vi "GetGlobalDefaultConfiguration.vi"(3 "Read defaults?":bool) -> (1 "Configuration File IV":path)   [LabVIEW 2013]
uses:
  MeasurementSetup.vi
panel:
  out "Configuration File Cis":path
  out "Configuration File Stability":path
  out "Configuration File CV":path
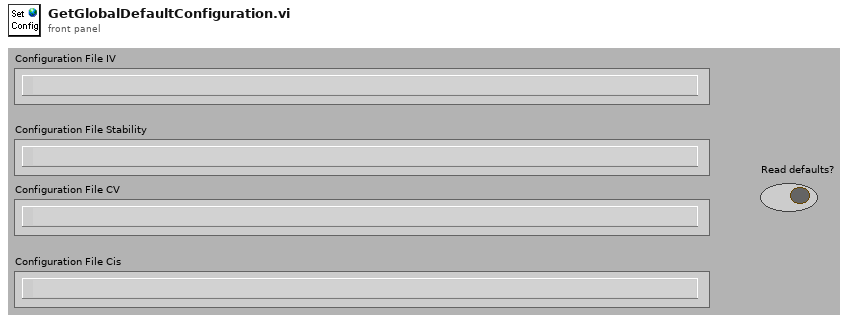
[diagram p1: front panel]
types:
  T1 = cluster{"Supply":refnum<class "SupplyControl.lvclass">, "Initial Voltage [V]":dbl, "Final Voltage [V]":dbl, "Step Size [V]":dbl, "Step Interval [s]":i32, "Number Of Steps":u32, "Ramp down steps [V]":dbl, "Ramp down Interval [s]":i32, "Set Current Limit?":bool, "Current Limit [µA]":dbl, "Temperature Readout":enum16{"Read Arduino", "Enter manually"}, "Arduino":refnum<class "ArduinoControl.lvclass">, "Supply Name":string}
  T2 = cluster{"Supply":refnum<class "SupplyControl.lvclass">, "LCR":refnum<class "LCRControl.lvclass">, "Initial Voltage [V]":dbl, "Final Voltage [V]":dbl, "Step Size [V]":dbl, "Step Interval [s]":i32, "Number Of Steps":u32, "AC frequency [Hz]":i32, "RC Configuration":u16, "AC amplitude [V]":dbl, "Ramp down steps [V]":dbl, "Ramp down Delay [s]":i32, "Set Current Limit?":bool, "Current Limit [µA]":dbl, "Temperature Readout":enum16{"Read Arduino", "Enter manually"}, "Arduino":refnum<class "ArduinoControl.lvclass">, "Supply Name":string, "LCR Name":string}
  T3 = cluster{"Supply":refnum<class "SupplyControl.lvclass">, "Voltage [V]":dbl, "Measurement Interval [s]":i32, "Test Duration":u32, "Ramp up steps [V]":dbl, "Ramp up Interval [s]":u32, "Ramp down steps [V]":dbl, "Ramp down Interval [s]":i32, "Set Current Limit?":bool, "Current Limit [µA]":dbl, "Temperature Readout":enum16{"Read Arduino", "Enter manually"}, "Arduino":refnum<class "ArduinoControl.lvclass">, "Supply Name":string}
  T4 = cluster{"Supply":refnum<class "SupplyControl.lvclass">, "LCR":refnum<class "LCRControl.lvclass">, "Initial Voltage [V]":dbl, "Final Voltage [V]":dbl, "Step Size [V]":dbl, "Step Interval [s]":i32, "Number Of Steps":u32, "AC frequency [Hz]":i32, "RC Configuration":u16, "AC amplitude [V]":dbl, "Ramp down steps [V]":dbl, "Ramp down Interval [s]":i32, "Set Current Limit?":bool, "Current Limit [µA]":dbl, "Temperature Readout":enum16{"Read Arduino", "Enter manually"}, "Arduino":refnum<class "ArduinoControl.lvclass">, "Supply Name":string, "LCR Name":string}
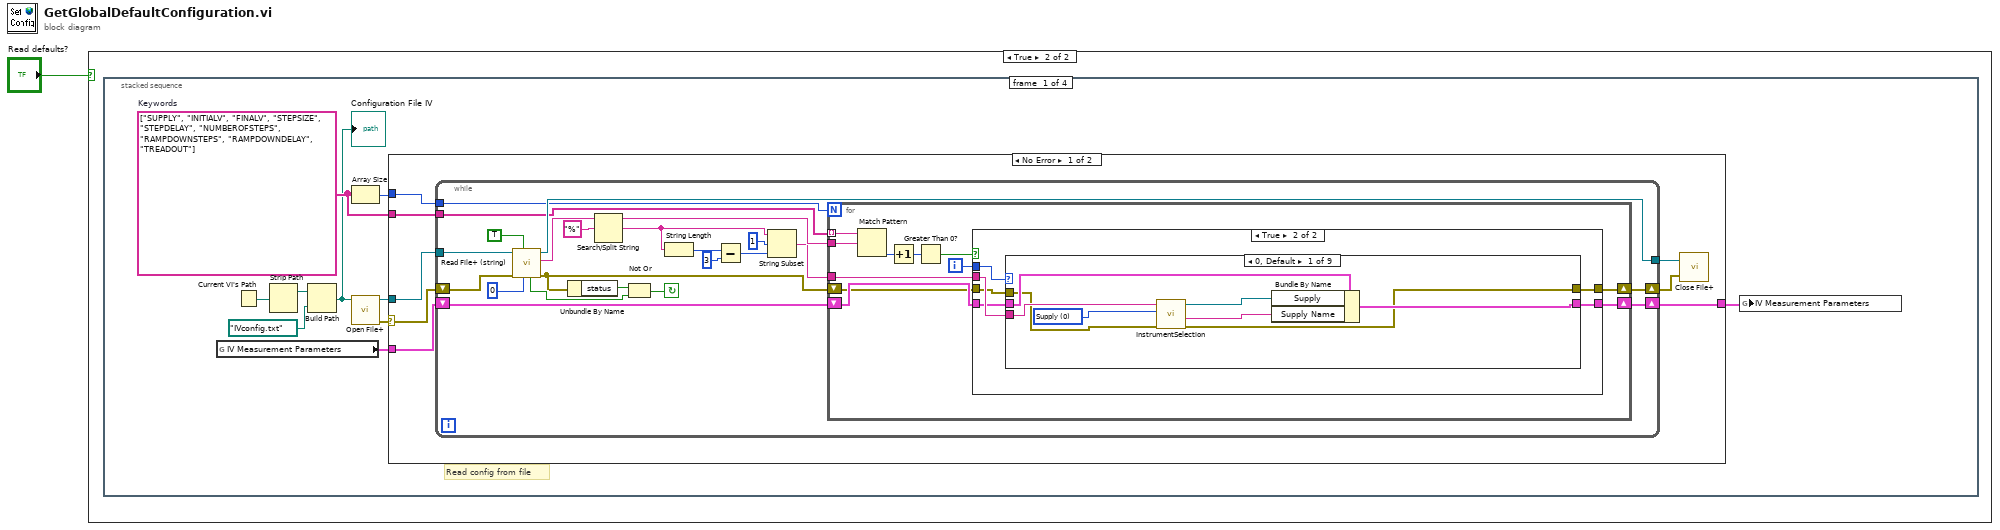
[diagram p0: block diagram]
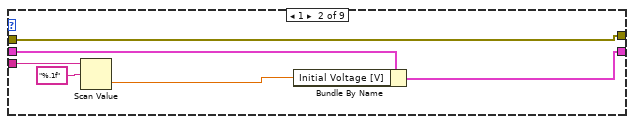
[diagram p4: hidden frame]
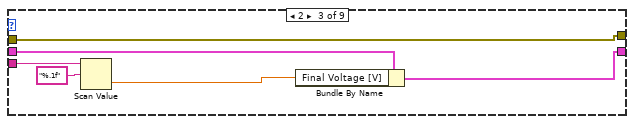
[diagram p5: hidden frame]
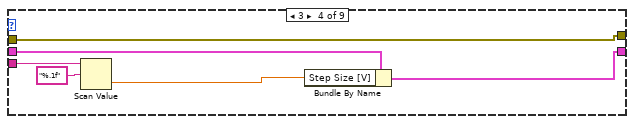
[diagram p6: hidden frame]
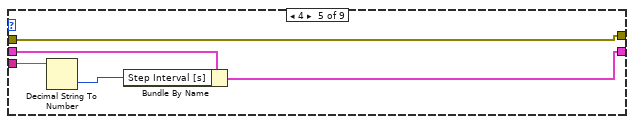
[diagram p7: hidden frame]
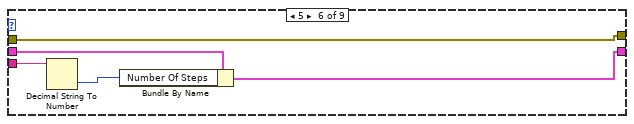
[diagram p8: hidden frame]
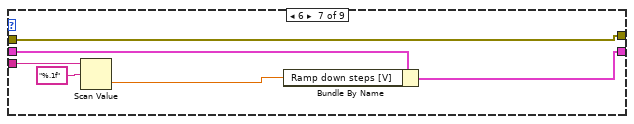
[diagram p9: hidden frame]
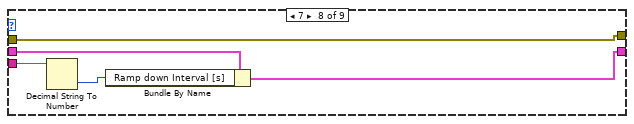
[diagram p10: hidden frame]
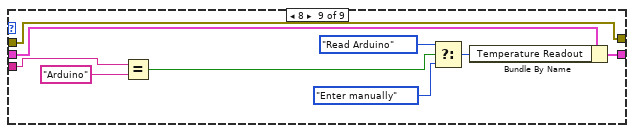
[diagram p11: hidden frame]
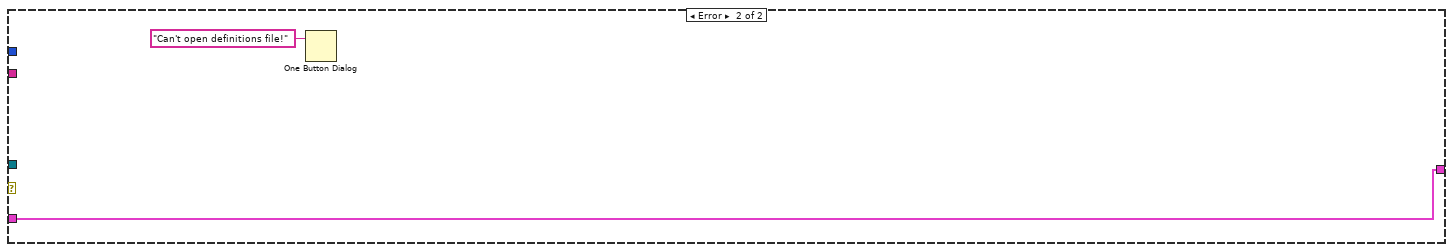
[diagram p12: hidden frame]
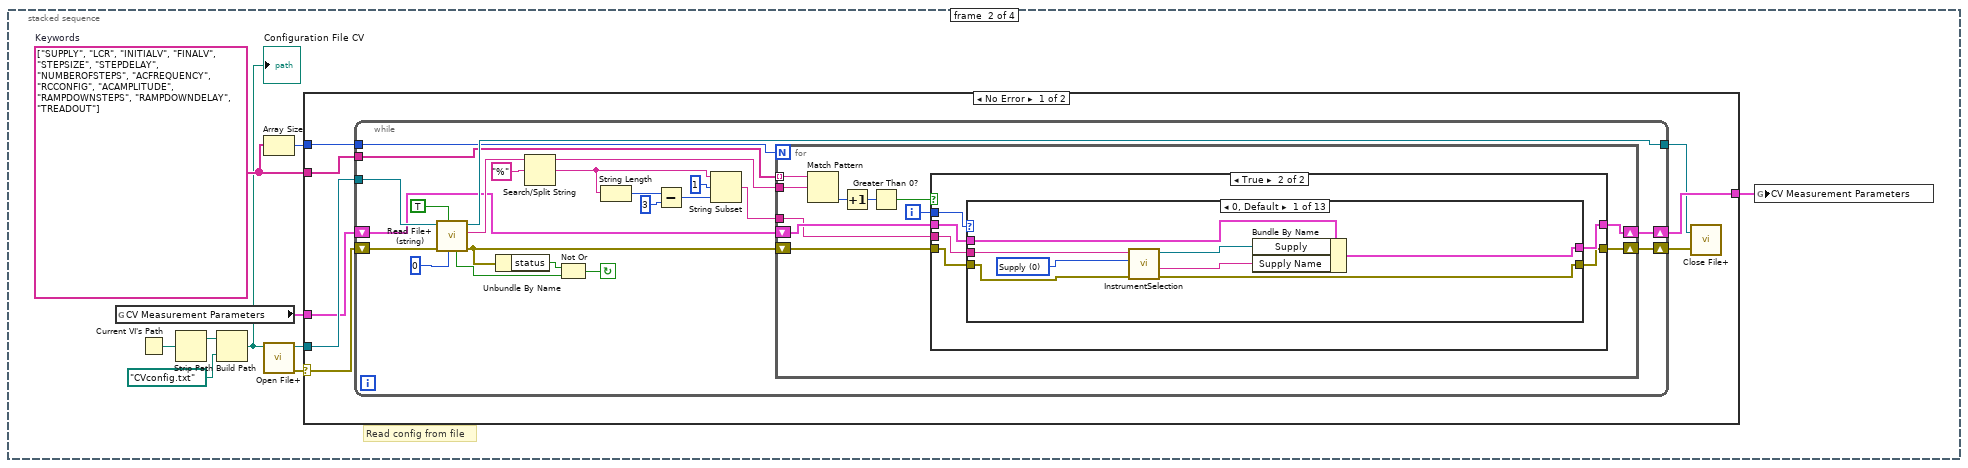
[diagram p13: hidden frame]
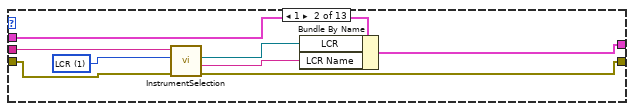
[diagram p15: hidden frame]
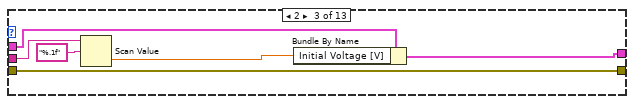
[diagram p16: hidden frame]
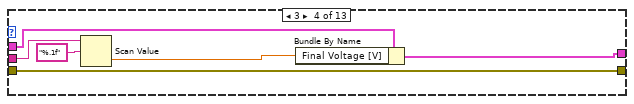
[diagram p17: hidden frame]
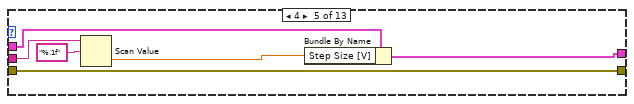
[diagram p18: hidden frame]
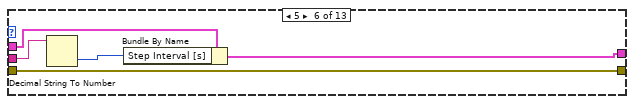
[diagram p19: hidden frame]
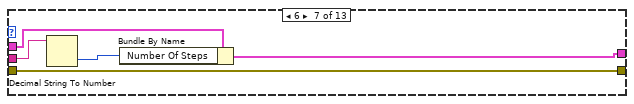
[diagram p20: hidden frame]
diagram:
  n1 = case shown="True" "Read defaults?" {
    frame False {
    }
    frame True {
      n2 = stacked-sequence {
        frame #0 {
          w11 = string[] ["SUPPLY", "INITIALV", "FINALV", "STEPSIZE", "STEPDELAY", "NUMBEROFSTEPS", "RAMPDOWNSTEPS", "RAMPDOWNDELAY", "TREADOUT"]  # Keywords
          # "Read config from file"
          n3 = global read "MeasurementSetup.vi" "IV Measurement Parameters"() -> (w2:T1)
          n4 = Current VI's Path() -> (path=w6:path)
          n5 = Strip Path(path=w6) -> (stripped path=w5:path)  [unwired: 1 out]
          n6 = Build Path(base path=w5, name or relative path=path "IVconfig.txt") -> (appended path=w4:path)
          "Configuration File IV" <- w4
          n7 = Array Size(array=w11) -> (size(s)=w10:i32)
          n8 = call <vilib>:"Open File+.vi"("file path (\" \")"=w4) -> ("error out"=w7:errorcluster, "refnum"=w8:refnum<file>)  [unwired: 7 in, 2 out]
          n9 = case shown="No Error" w7 {
            selector: w7 -> [w12 _]
            tunnel: w8 -> [w19 _]
            tunnel: w11 -> [w18 _]
            tunnel: w10 -> [w17 _]
            tunnel: w2 -> [w16 w118]
            tunnel: [w15 w118] -> w3
            frame No Error {
              n10 = while {
                shift-left: w16 -> [w25]
                shift-right: [w23] -> w15
                tunnel: w17 -> [w22]
                tunnel: w18 -> [w28]
                tunnel: [w33] -> w14
                tunnel: w19 -> [w39]
                shift-right: [w20] -> w13
                shift-left: w12 -> [w32]
                stop <- w35 continue-if-true
                n11 = call <vilib>:"Read File+ (string).vi"("count"=0, "line mode (characters:F)"=TRUE, "error in (no error)"=w32, "refnum"=w39) -> ("error out"=w21:errorcluster, "string"=w34:string, "dup refnum"=w33:refnum<file>, "EOF?"=w37:bool)  [unwired: 3 in, 1 out]
                n12 = Unbundle By Name(w21) -> ("status"=w36:bool)
                n13 = Search/Split String(string=w34, search string/char (-)="%" ("search char (-)")) -> (substring before match=w27:string, match + rest of string=w40:string)  [unwired: 1 in, 1 out]
                n14 = Not Or(1:w37, 2:w36) -> (0:w35:bool)
                n15 = String Length(string=w40) -> (length=w26:i32)
                n16 = Subtract(x=w26, y=3) -> (x-y=w29:i32)
                n17 = String Subset(string=w40, offset (0)=1, length (rest)=w29) -> (substring=w24:string)
                n18 = for {
                  N: w22 -> [_]
                  tunnel: w28 -> [w51] mode=indexing
                  tunnel: w27 -> [w46]
                  shift-right: [w47] -> w23
                  shift-left: w25 -> [w48]
                  tunnel: w24 -> [w45]
                  shift-right: [w43] -> w20
                  shift-left: w21 -> [w44]
                  i -> [w49]
                  n19 = Match Pattern(string=w51, regular expression=w46) -> (offset past match=w52:i32)  [unwired: 1 in, 3 out]
                  n20 = Increment(x=w52) -> (x+1=w53:i32)
                  n21 = Greater Than 0?(x=w53) -> (x > 0?=w50:bool)
                  n22 = case shown="True" w50 {
                    tunnel: w49 -> [_ w61]
                    tunnel: w45 -> [_ w60]
                    tunnel: w48 -> [w55 w59]
                    tunnel: [w55 w58] -> w47
                    tunnel: w44 -> [w54 w57]
                    tunnel: [w54 w56] -> w43
                    frame False {
                    }
                    frame True {
                      n23 = case shown="0, Default" w61 {
                        tunnel: w60 -> [w66 w73 w78 w84 w90 w95 w100 w106 w115]
                        tunnel: w59 -> [w69 w75 w81 w87 w92 w97 w103 w108 w117]
                        tunnel: [w68 w74 w80 w86 w91 w96 w102 w107 w116] -> w58
                        tunnel: w57 -> [w65 w70 w76 w82 w88 w93 w98 w104 w109]
                        tunnel: [w64 w70 w76 w82 w88 w93 w98 w104 w109] -> w56
                        frame 0, Default {
                          w67 = u16 0 items=["Supply", "LCR"] ("Instrument type")
                          n24 = call "InstrumentSelection.vi"("error in (no error)"=w65, "Instrument type"=w67, "Instrument name IN"=w66) -> ("error out"=w64:errorcluster, "Instrument name OUT"=w63:string, "Supply"=w62:refnum<class "SupplyControl.lvclass">)  [unwired: 5 in, 1 out]
                          n25 = Bundle By Name(cluster=w69, "Supply"=w62, "Supply Name"=w63) -> (w68:T1)
                        }
                        frame 1 {
                          n26 = Scan Value(string=w73, format string="%.1f") -> (value=w72:dbl)  [unwired: 1 in, 1 out]
                          n27 = Bundle By Name(cluster=w75, "Initial Voltage [V]"=w72) -> (w74:T1)
                        }
                        frame 2 {
                          n28 = Scan Value(string=w78, format string="%.1f") -> (value=w77:dbl)  [unwired: 1 in, 1 out]
                          n29 = Bundle By Name(cluster=w81, "Final Voltage [V]"=w77) -> (w80:T1)
                        }
                        frame 3 {
                          n30 = Scan Value(string=w84, format string="%.1f") -> (value=w83:dbl)  [unwired: 1 in, 1 out]
                          n31 = Bundle By Name(cluster=w87, "Step Size [V]"=w83) -> (w86:T1)
                        }
                        frame 4 {
                          n32 = Decimal String To Number(string=w90) -> (number=w89:i32)  [unwired: 2 in, 1 out]
                          n33 = Bundle By Name(cluster=w92, "Step Interval [s]"=w89) -> (w91:T1)
                        }
                        frame 5 {
                          n34 = Decimal String To Number(string=w95) -> (number=w94:i32)  [unwired: 2 in, 1 out]
                          n35 = Bundle By Name(cluster=w97, "Number Of Steps"=w94) -> (w96:T1)
                        }
                        frame 6 {
                          n36 = Scan Value(string=w100, format string="%.1f") -> (value=w99:dbl)  [unwired: 1 in, 1 out]
                          n37 = Bundle By Name(cluster=w103, "Ramp down steps [V]"=w99) -> (w102:T1)
                        }
                        frame 7 {
                          n38 = Decimal String To Number(string=w106) -> (number=w105:i32)  [unwired: 2 in, 1 out]
                          n39 = Bundle By Name(cluster=w108, "Ramp down Interval [s]"=w105) -> (w107:T1)
                        }
                        frame 8 {
                          n40 = Equal?(x=w115, y="Arduino") -> (x = y?=w113:bool)
                          n41 = Select(t=enum16{"Read Arduino", "Enter manually"}."Read Arduino" ("Temperature Readout"), s=w113, f=enum16{"Read Arduino", "Enter manually"}."Enter manually" ("Temperature Readout")) -> (s? t:f=w110:enum16{"Read Arduino", "Enter manually"})
                          n42 = Bundle By Name(cluster=w117, "Temperature Readout"=w110) -> (w116:T1)
                        }
                      }
                    }
                  }
                }
              }
              n43 = call <vilib>:"Close File+.vi"("error in (no error)"=w13, "refnum"=w14) -> ()  [unwired: 3 in, 3 out]
            }
            frame Error {
              n44 = One Button Dialog(message="Can't open definitions file!") -> ()  [unwired: 1 in, 1 out]
            }
          }
          n45 = global write "MeasurementSetup.vi" "IV Measurement Parameters"(w3) -> ()
        }
        frame #1 {
          w129 = string[] ["SUPPLY", "LCR", "INITIALV", "FINALV", "STEPSIZE", "STEPDELAY", "NUMBEROFSTEPS", "ACFREQUENCY", "RCCONFIG", "ACAMPLITUDE", "RAMPDOWNSTEPS", "RAMPDOWNDELAY", "TREADOUT"]  # Keywords
          # "Read config from file"
          n46 = global read "MeasurementSetup.vi" "CV Measurement Parameters"() -> (w120:T2)
          n47 = Current VI's Path() -> (path=w124:path)
          n48 = Strip Path(path=w124) -> (stripped path=w123:path)  [unwired: 1 out]
          n49 = Build Path(base path=w123, name or relative path=path "CVconfig.txt") -> (appended path=w122:path)
          "Configuration File CV" <- w122
          n50 = Array Size(array=w129) -> (size(s)=w128:i32)
          n51 = call <vilib>:"Open File+.vi"("file path (\" \")"=w122) -> ("error out"=w125:errorcluster, "refnum"=w126:refnum<file>)  [unwired: 7 in, 2 out]
          n52 = case shown="No Error" w125 {
            selector: w125 -> [w130 _]
            tunnel: w126 -> [w137 _]
            tunnel: w129 -> [w136 _]
            tunnel: w128 -> [w135 _]
            tunnel: w120 -> [w134 w264]
            tunnel: [w133 w264] -> w121
            frame No Error {
              n53 = while {
                shift-left: w134 -> [w143]
                shift-right: [w141] -> w133
                tunnel: w135 -> [w140]
                tunnel: w136 -> [w146]
                tunnel: [w151] -> w132
                tunnel: w137 -> [w157]
                shift-right: [w138] -> w131
                shift-left: w130 -> [w150]
                stop <- w153 continue-if-true
                n54 = call <vilib>:"Read File+ (string).vi"("count"=0, "line mode (characters:F)"=TRUE, "error in (no error)"=w150, "refnum"=w157) -> ("error out"=w139:errorcluster, "string"=w152:string, "dup refnum"=w151:refnum<file>, "EOF?"=w155:bool)  [unwired: 3 in, 1 out]
                n55 = Unbundle By Name(w139) -> ("status"=w154:bool)
                n56 = Search/Split String(string=w152, search string/char (-)="%" ("search char (-)")) -> (substring before match=w145:string, match + rest of string=w158:string)  [unwired: 1 in, 1 out]
                n57 = Not Or(1:w155, 2:w154) -> (0:w153:bool)
                n58 = String Length(string=w158) -> (length=w144:i32)
                n59 = Subtract(x=w144, y=3) -> (x-y=w147:i32)
                n60 = String Subset(string=w158, offset (0)=1, length (rest)=w147) -> (substring=w142:string)
                n61 = for {
                  N: w140 -> [_]
                  tunnel: w146 -> [w169] mode=indexing
                  tunnel: w145 -> [w164]
                  shift-right: [w165] -> w141
                  shift-left: w143 -> [w166]
                  tunnel: w142 -> [w163]
                  shift-right: [w161] -> w138
                  shift-left: w139 -> [w162]
                  i -> [w167]
                  n62 = Match Pattern(string=w169, regular expression=w164) -> (offset past match=w170:i32)  [unwired: 1 in, 3 out]
                  n63 = Increment(x=w170) -> (x+1=w171:i32)
                  n64 = Greater Than 0?(x=w171) -> (x > 0?=w168:bool)
                  n65 = case shown="True" w168 {
                    tunnel: w167 -> [_ w179]
                    tunnel: w163 -> [_ w178]
                    tunnel: w166 -> [w173 w177]
                    tunnel: [w173 w176] -> w165
                    tunnel: w162 -> [w172 w175]
                    tunnel: [w172 w174] -> w161
                    frame False {
                    }
                    frame True {
                      n66 = case shown="0, Default" w179 {
                        tunnel: w178 -> [w183 w191 w199 w204 w210 w216 w221 w226 w234 w243 w246 w252 w261]
                        tunnel: w177 -> [w187 w195 w201 w207 w213 w218 w223 w228 w237 w241 w249 w254 w263]
                        tunnel: [w186 w194 w200 w206 w212 w217 w222 w227 w236 w239 w248 w253 w262] -> w176
                        tunnel: w175 -> [w184 w193 w196 w202 w208 w214 w219 w224 w229 w238 w244 w250 w255]
                        tunnel: [w185 w192 w196 w202 w208 w214 w219 w224 w229 w238 w244 w250 w255] -> w174
                        frame 0, Default {
                          w182 = u16 0 items=["Supply", "LCR"] ("Instrument type")
                          n67 = call "InstrumentSelection.vi"("error in (no error)"=w184, "Instrument type"=w182, "Instrument name IN"=w183) -> ("error out"=w185:errorcluster, "Instrument name OUT"=w180:string, "Supply"=w181:refnum<class "SupplyControl.lvclass">)  [unwired: 5 in, 1 out]
                          n68 = Bundle By Name(cluster=w187, "Supply"=w181, "Supply Name"=w180) -> (w186:T2)
                        }
                        frame 1 {
                          w190 = u16 1 items=["Supply", "LCR"] ("Instrument type")
                          n69 = call "InstrumentSelection.vi"("error in (no error)"=w193, "Instrument type"=w190, "Instrument name IN"=w191) -> ("error out"=w192:errorcluster, "Instrument name OUT"=w189:string, "LCR"=w188:refnum<class "LCRControl.lvclass">)  [unwired: 5 in, 1 out]
                          n70 = Bundle By Name(cluster=w195, "LCR"=w188, "LCR Name"=w189) -> (w194:T2)
                        }
                        frame 2 {
                          n71 = Scan Value(string=w199, format string="%.1f") -> (value=w198:dbl)  [unwired: 1 in, 1 out]
                          n72 = Bundle By Name(cluster=w201, "Initial Voltage [V]"=w198) -> (w200:T2)
                        }
                        frame 3 {
                          n73 = Scan Value(string=w204, format string="%.1f") -> (value=w203:dbl)  [unwired: 1 in, 1 out]
                          n74 = Bundle By Name(cluster=w207, "Final Voltage [V]"=w203) -> (w206:T2)
                        }
                        frame 4 {
                          n75 = Scan Value(string=w210, format string="%.1f") -> (value=w209:dbl)  [unwired: 1 in, 1 out]
                          n76 = Bundle By Name(cluster=w213, "Step Size [V]"=w209) -> (w212:T2)
                        }
                        frame 5 {
                          n77 = Decimal String To Number(string=w216) -> (number=w215:i32)  [unwired: 2 in, 1 out]
                          n78 = Bundle By Name(cluster=w218, "Step Interval [s]"=w215) -> (w217:T2)
                        }
                        frame 6 {
                          n79 = Decimal String To Number(string=w221) -> (number=w220:i32)  [unwired: 2 in, 1 out]
                          n80 = Bundle By Name(cluster=w223, "Number Of Steps"=w220) -> (w222:T2)
                        }
                        frame 7 {
                          n81 = Decimal String To Number(string=w226) -> (number=w225:i32)  [unwired: 2 in, 1 out]
                          n82 = Bundle By Name(cluster=w228, "AC frequency [Hz]"=w225) -> (w227:T2)
                        }
                        frame 8 {
                          w233 = u16 0 items=["serial", "parallel"] ("RC Configuration")
                          w232 = u16 1 items=["serial", "parallel"] ("RC Configuration")
                          n83 = Equal?(x=w234, y="serial") -> (x = y?=w231:bool)
                          n84 = Select(t=w233, s=w231, f=w232) -> (s? t:f=w230:u16)
                          n85 = Bundle By Name(cluster=w237, "RC Configuration"=w230) -> (w236:T2)
                        }
                        frame 9 {
                          n86 = Scan Value(string=w243, format string="%.1f") -> (value=w240:dbl)  [unwired: 1 in, 1 out]
                          n87 = Bundle By Name(cluster=w241, "AC amplitude [V]"=w240) -> (w239:T2)
                        }
                        frame 10 {
                          n88 = Scan Value(string=w246, format string="%.1f") -> (value=w245:dbl)  [unwired: 1 in, 1 out]
                          n89 = Bundle By Name(cluster=w249, "Ramp down steps [V]"=w245) -> (w248:T2)
                        }
                        frame 11 {
                          n90 = Decimal String To Number(string=w252) -> (number=w251:i32)  [unwired: 2 in, 1 out]
                          n91 = Bundle By Name(cluster=w254, "Ramp down Delay [s]"=w251) -> (w253:T2)
                        }
                        frame 12 {
                          n92 = Equal?(x=w261, y="Arduino") -> (x = y?=w259:bool)
                          n93 = Select(t=enum16{"Read Arduino", "Enter manually"}."Read Arduino" ("Temperature Readout"), s=w259, f=enum16{"Read Arduino", "Enter manually"}."Enter manually" ("Temperature Readout")) -> (s? t:f=w256:enum16{"Read Arduino", "Enter manually"})
                          n94 = Bundle By Name(cluster=w263, "Temperature Readout"=w256) -> (w262:T2)
                        }
                      }
                    }
                  }
                }
              }
              n95 = call <vilib>:"Close File+.vi"("error in (no error)"=w131, "refnum"=w132) -> ()  [unwired: 3 in, 3 out]
            }
            frame Error {
              n96 = One Button Dialog(message="Can't open definitions file!") -> ()  [unwired: 1 in, 1 out]
            }
          }
          n97 = global write "MeasurementSetup.vi" "CV Measurement Parameters"(w121) -> ()
        }
        frame #2 {
          w275 = string[] ["SUPPLY", "VOLTAGE", "INTERVAL", "DURATION", "RAMPUPSTEPS", "RAMPUPDELAY", "RAMPDOWNSTEPS", "RAMPDOWNDELAY", "TREADOUT"]  # Keywords
          # "Read config from file"
          n98 = global read "MeasurementSetup.vi" "Current Stability Measurement Parameters"() -> (w266:T3)
          n99 = Current VI's Path() -> (path=w270:path)
          n100 = Strip Path(path=w270) -> (stripped path=w269:path)  [unwired: 1 out]
          n101 = Build Path(base path=w269, name or relative path=path "STABILITYconfig.txt") -> (appended path=w268:path)
          "Configuration File Stability" <- w268
          n102 = Array Size(array=w275) -> (size(s)=w274:i32)
          n103 = call <vilib>:"Open File+.vi"("file path (\" \")"=w268) -> ("error out"=w271:errorcluster, "refnum"=w272:refnum<file>)  [unwired: 7 in, 2 out]
          n104 = case shown="No Error" w271 {
            selector: w271 -> [w276 _]
            tunnel: w272 -> [w283 _]
            tunnel: w275 -> [w282 _]
            tunnel: w274 -> [w281 _]
            tunnel: w266 -> [w280 w381]
            tunnel: [w279 w381] -> w267
            frame No Error {
              n105 = while {
                shift-left: w280 -> [w289]
                shift-right: [w287] -> w279
                tunnel: w281 -> [w286]
                tunnel: w282 -> [w292]
                tunnel: [w297] -> w278
                tunnel: w283 -> [w303]
                shift-right: [w284] -> w277
                shift-left: w276 -> [w296]
                stop <- w299 continue-if-true
                n106 = call <vilib>:"Read File+ (string).vi"("count"=0, "line mode (characters:F)"=TRUE, "error in (no error)"=w296, "refnum"=w303) -> ("error out"=w285:errorcluster, "string"=w298:string, "dup refnum"=w297:refnum<file>, "EOF?"=w301:bool)  [unwired: 3 in, 1 out]
                n107 = Unbundle By Name(w285) -> ("status"=w300:bool)
                n108 = Search/Split String(string=w298, search string/char (-)="%" ("search char (-)")) -> (substring before match=w291:string, match + rest of string=w304:string)  [unwired: 1 in, 1 out]
                n109 = Not Or(1:w301, 2:w300) -> (0:w299:bool)
                n110 = String Length(string=w304) -> (length=w290:i32)
                n111 = Subtract(x=w290, y=3) -> (x-y=w293:i32)
                n112 = String Subset(string=w304, offset (0)=1, length (rest)=w293) -> (substring=w288:string)
                n113 = for {
                  N: w286 -> [_]
                  tunnel: w292 -> [w315] mode=indexing
                  tunnel: w291 -> [w310]
                  shift-right: [w311] -> w287
                  shift-left: w289 -> [w312]
                  tunnel: w288 -> [w309]
                  shift-right: [w307] -> w284
                  shift-left: w285 -> [w308]
                  i -> [w313]
                  n114 = Match Pattern(string=w315, regular expression=w310) -> (offset past match=w316:i32)  [unwired: 1 in, 3 out]
                  n115 = Increment(x=w316) -> (x+1=w317:i32)
                  n116 = Greater Than 0?(x=w317) -> (x > 0?=w314:bool)
                  n117 = case shown="True" w314 {
                    tunnel: w313 -> [_ w325]
                    tunnel: w309 -> [_ w324]
                    tunnel: w312 -> [w319 w323]
                    tunnel: [w319 w322] -> w311
                    tunnel: w308 -> [w318 w321]
                    tunnel: [w318 w320] -> w307
                    frame False {
                    }
                    frame True {
                      n118 = case shown="0, Default" w325 {
                        tunnel: w324 -> [w330 w337 w341 w346 w352 w358 w363 w369 w378]
                        tunnel: w323 -> [w333 w339 w344 w349 w355 w360 w366 w371 w380]
                        tunnel: [w332 w338 w343 w348 w354 w359 w365 w370 w379] -> w322
                        tunnel: w321 -> [w329 w334 w342 w347 w353 w356 w361 w367 w372]
                        tunnel: [w328 w334 w342 w347 w353 w356 w361 w367 w372] -> w320
                        frame 0, Default {
                          w331 = u16 0 items=["Supply", "LCR"] ("Instrument type")
                          n119 = call "InstrumentSelection.vi"("error in (no error)"=w329, "Instrument type"=w331, "Instrument name IN"=w330) -> ("error out"=w328:errorcluster, "Instrument name OUT"=w327:string, "Supply"=w326:refnum<class "SupplyControl.lvclass">)  [unwired: 5 in, 1 out]
                          n120 = Bundle By Name(cluster=w333, "Supply"=w326, "Supply Name"=w327) -> (w332:T3)
                        }
                        frame 1 {
                          n121 = Scan Value(string=w337, format string="%.1f") -> (value=w336:dbl)  [unwired: 1 in, 1 out]
                          n122 = Bundle By Name(cluster=w339, "Voltage [V]"=w336) -> (w338:T3)
                        }
                        frame 2 {
                          n123 = Decimal String To Number(string=w341) -> (number=w340:i32)  [unwired: 2 in, 1 out]
                          n124 = Bundle By Name(cluster=w344, "Measurement Interval [s]"=w340) -> (w343:T3)
                        }
                        frame 3 {
                          n125 = Decimal String To Number(string=w346) -> (number=w345:i32)  [unwired: 2 in, 1 out]
                          n126 = Bundle By Name(cluster=w349, "Test Duration"=w345) -> (w348:T3)
                        }
                        frame 4 {
                          n127 = Scan Value(string=w352, format string="%.1f") -> (value=w350:dbl)  [unwired: 1 in, 1 out]
                          n128 = Bundle By Name(cluster=w355, "Ramp up steps [V]"=w350) -> (w354:T3)
                        }
                        frame 5 {
                          n129 = Decimal String To Number(string=w358) -> (number=w357:i32)  [unwired: 2 in, 1 out]
                          n130 = Bundle By Name(cluster=w360, "Ramp up Interval [s]"=w357) -> (w359:T3)
                        }
                        frame 6 {
                          n131 = Scan Value(string=w363, format string="%.1f") -> (value=w362:dbl)  [unwired: 1 in, 1 out]
                          n132 = Bundle By Name(cluster=w366, "Ramp down steps [V]"=w362) -> (w365:T3)
                        }
                        frame 7 {
                          n133 = Decimal String To Number(string=w369) -> (number=w368:i32)  [unwired: 2 in, 1 out]
                          n134 = Bundle By Name(cluster=w371, "Ramp down Interval [s]"=w368) -> (w370:T3)
                        }
                        frame 8 {
                          n135 = Equal?(x=w378, y="Arduino") -> (x = y?=w376:bool)
                          n136 = Select(t=enum16{"Read Arduino", "Enter manually"}."Read Arduino" ("Temperature Readout"), s=w376, f=enum16{"Read Arduino", "Enter manually"}."Enter manually" ("Temperature Readout")) -> (s? t:f=w373:enum16{"Read Arduino", "Enter manually"})
                          n137 = Bundle By Name(cluster=w380, "Temperature Readout"=w373) -> (w379:T3)
                        }
                      }
                    }
                  }
                }
              }
              n138 = call <vilib>:"Close File+.vi"("error in (no error)"=w277, "refnum"=w278) -> ()  [unwired: 3 in, 3 out]
            }
            frame Error {
              n139 = One Button Dialog(message="Can't open definitions file!") -> ()  [unwired: 1 in, 1 out]
            }
          }
          n140 = global write "MeasurementSetup.vi" "Current Stability Measurement Parameters"(w267) -> ()
        }
        frame #3 {
          w392 = string[] ["SUPPLY", "LCR", "INITIALV", "FINALV", "STEPSIZE", "STEPDELAY", "NUMBEROFSTEPS", "ACFREQUENCY", "RCCONFIG", "ACAMPLITUDE", "RAMPDOWNSTEPS", "RAMPDOWNDELAY", "TREADOUT"]  # Keywords
          # "Read config from file"
          n141 = global read "MeasurementSetup.vi" "Cis Measurement Parameters"() -> (w383:T4)
          n142 = Current VI's Path() -> (path=w387:path)
          n143 = Strip Path(path=w387) -> (stripped path=w386:path)  [unwired: 1 out]
          n144 = Build Path(base path=w386, name or relative path=path "CISconfig.txt") -> (appended path=w385:path)
          "Configuration File Cis" <- w385
          n145 = Array Size(array=w392) -> (size(s)=w391:i32)
          n146 = call <vilib>:"Open File+.vi"("file path (\" \")"=w385) -> ("error out"=w388:errorcluster, "refnum"=w389:refnum<file>)  [unwired: 7 in, 2 out]
          n147 = case shown="No Error" w388 {
            selector: w388 -> [w393 _]
            tunnel: w389 -> [w400 _]
            tunnel: w392 -> [w399 _]
            tunnel: w391 -> [w398 _]
            tunnel: w383 -> [w397 w527]
            tunnel: [w396 w527] -> w384
            frame No Error {
              n148 = while {
                shift-left: w397 -> [w406]
                shift-right: [w404] -> w396
                tunnel: w398 -> [w403]
                tunnel: w399 -> [w409]
                tunnel: [w414] -> w395
                tunnel: w400 -> [w420]
                shift-right: [w401] -> w394
                shift-left: w393 -> [w413]
                stop <- w416 continue-if-true
                n149 = call <vilib>:"Read File+ (string).vi"("count"=0, "line mode (characters:F)"=TRUE, "error in (no error)"=w413, "refnum"=w420) -> ("error out"=w402:errorcluster, "string"=w415:string, "dup refnum"=w414:refnum<file>, "EOF?"=w418:bool)  [unwired: 3 in, 1 out]
                n150 = Unbundle By Name(w402) -> ("status"=w417:bool)
                n151 = Search/Split String(string=w415, search string/char (-)="%" ("search char (-)")) -> (substring before match=w408:string, match + rest of string=w421:string)  [unwired: 1 in, 1 out]
                n152 = Not Or(1:w418, 2:w417) -> (0:w416:bool)
                n153 = String Length(string=w421) -> (length=w407:i32)
                n154 = Subtract(x=w407, y=3) -> (x-y=w410:i32)
                n155 = String Subset(string=w421, offset (0)=1, length (rest)=w410) -> (substring=w405:string)
                n156 = for {
                  N: w403 -> [_]
                  tunnel: w409 -> [w432] mode=indexing
                  tunnel: w408 -> [w427]
                  shift-right: [w428] -> w404
                  shift-left: w406 -> [w429]
                  tunnel: w405 -> [w426]
                  shift-right: [w424] -> w401
                  shift-left: w402 -> [w425]
                  i -> [w430]
                  n157 = Match Pattern(string=w432, regular expression=w427) -> (offset past match=w433:i32)  [unwired: 1 in, 3 out]
                  n158 = Increment(x=w433) -> (x+1=w434:i32)
                  n159 = Greater Than 0?(x=w434) -> (x > 0?=w431:bool)
                  n160 = case shown="True" w431 {
                    tunnel: w430 -> [_ w442]
                    tunnel: w426 -> [_ w441]
                    tunnel: w429 -> [w436 w440]
                    tunnel: [w436 w439] -> w428
                    tunnel: w425 -> [w435 w438]
                    tunnel: [w435 w437] -> w424
                    frame False {
                    }
                    frame True {
                      n161 = case shown="0, Default" w442 {
                        tunnel: w441 -> [w446 w454 w462 w467 w473 w479 w484 w489 w497 w506 w509 w515 w524]
                        tunnel: w440 -> [w450 w458 w464 w470 w476 w481 w486 w491 w500 w504 w512 w517 w526]
                        tunnel: [w449 w457 w463 w469 w475 w480 w485 w490 w499 w502 w511 w516 w525] -> w439
                        tunnel: w438 -> [w447 w456 w459 w465 w471 w477 w482 w487 w492 w501 w507 w513 w518]
                        tunnel: [w448 w455 w459 w465 w471 w477 w482 w487 w492 w501 w507 w513 w518] -> w437
                        frame 0, Default {
                          w445 = u16 0 items=["Supply", "LCR"] ("Instrument type")
                          n162 = call "InstrumentSelection.vi"("error in (no error)"=w447, "Instrument type"=w445, "Instrument name IN"=w446) -> ("error out"=w448:errorcluster, "Instrument name OUT"=w443:string, "Supply"=w444:refnum<class "SupplyControl.lvclass">)  [unwired: 5 in, 1 out]
                          n163 = Bundle By Name(cluster=w450, "Supply"=w444, "Supply Name"=w443) -> (w449:T4)
                        }
                        frame 1 {
                          w453 = u16 1 items=["Supply", "LCR"] ("Instrument type")
                          n164 = call "InstrumentSelection.vi"("error in (no error)"=w456, "Instrument type"=w453, "Instrument name IN"=w454) -> ("error out"=w455:errorcluster, "Instrument name OUT"=w452:string, "LCR"=w451:refnum<class "LCRControl.lvclass">)  [unwired: 5 in, 1 out]
                          n165 = Bundle By Name(cluster=w458, "LCR"=w451, "LCR Name"=w452) -> (w457:T4)
                        }
                        frame 2 {
                          n166 = Scan Value(string=w462, format string="%.1f") -> (value=w461:dbl)  [unwired: 1 in, 1 out]
                          n167 = Bundle By Name(cluster=w464, "Initial Voltage [V]"=w461) -> (w463:T4)
                        }
                        frame 3 {
                          n168 = Scan Value(string=w467, format string="%.1f") -> (value=w466:dbl)  [unwired: 1 in, 1 out]
                          n169 = Bundle By Name(cluster=w470, "Final Voltage [V]"=w466) -> (w469:T4)
                        }
                        frame 4 {
                          n170 = Scan Value(string=w473, format string="%.1f") -> (value=w472:dbl)  [unwired: 1 in, 1 out]
                          n171 = Bundle By Name(cluster=w476, "Step Size [V]"=w472) -> (w475:T4)
                        }
                        frame 5 {
                          n172 = Decimal String To Number(string=w479) -> (number=w478:i32)  [unwired: 2 in, 1 out]
                          n173 = Bundle By Name(cluster=w481, "Step Interval [s]"=w478) -> (w480:T4)
                        }
                        frame 6 {
                          n174 = Decimal String To Number(string=w484) -> (number=w483:i32)  [unwired: 2 in, 1 out]
                          n175 = Bundle By Name(cluster=w486, "Number Of Steps"=w483) -> (w485:T4)
                        }
                        frame 7 {
                          n176 = Decimal String To Number(string=w489) -> (number=w488:i32)  [unwired: 2 in, 1 out]
                          n177 = Bundle By Name(cluster=w491, "AC frequency [Hz]"=w488) -> (w490:T4)
                        }
                        frame 8 {
                          w496 = u16 0 items=["serial", "parallel"] ("RC Configuration")
                          w495 = u16 1 items=["serial", "parallel"] ("RC Configuration")
                          n178 = Equal?(x=w497, y="serial") -> (x = y?=w494:bool)
                          n179 = Select(t=w496, s=w494, f=w495) -> (s? t:f=w493:u16)
                          n180 = Bundle By Name(cluster=w500, "RC Configuration"=w493) -> (w499:T4)
                        }
                        frame 9 {
                          n181 = Scan Value(string=w506, format string="%.1f") -> (value=w503:dbl)  [unwired: 1 in, 1 out]
                          n182 = Bundle By Name(cluster=w504, "AC amplitude [V]"=w503) -> (w502:T4)
                        }
                        frame 10 {
                          n183 = Scan Value(string=w509, format string="%.1f") -> (value=w508:dbl)  [unwired: 1 in, 1 out]
                          n184 = Bundle By Name(cluster=w512, "Ramp down steps [V]"=w508) -> (w511:T4)
                        }
                        frame 11 {
                          n185 = Decimal String To Number(string=w515) -> (number=w514:i32)  [unwired: 2 in, 1 out]
                          n186 = Bundle By Name(cluster=w517, "Ramp down Interval [s]"=w514) -> (w516:T4)
                        }
                        frame 12 {
                          n187 = Equal?(x=w524, y="Arduino") -> (x = y?=w522:bool)
                          n188 = Select(t=enum16{"Read Arduino", "Enter manually"}."Read Arduino" ("Temperature Readout"), s=w522, f=enum16{"Read Arduino", "Enter manually"}."Enter manually" ("Temperature Readout")) -> (s? t:f=w519:enum16{"Read Arduino", "Enter manually"})
                          n189 = Bundle By Name(cluster=w526, "Temperature Readout"=w519) -> (w525:T4)
                        }
                      }
                    }
                  }
                }
              }
              n190 = call <vilib>:"Close File+.vi"("error in (no error)"=w394, "refnum"=w395) -> ()  [unwired: 3 in, 3 out]
            }
            frame Error {
              n191 = One Button Dialog(message="Can't open definitions file!") -> ()  [unwired: 1 in, 1 out]
            }
          }
          n192 = global write "MeasurementSetup.vi" "Cis Measurement Parameters"(w384) -> ()
        }
      }
    }
  }
